vi "Galvo-Control-V3.vi"() -> ()   [LabVIEW 2024]
uses:
  <vilib>/DAQmx/write.llb/DAQmx Write (Analog 2D DBL NChan NSamp).vi
  <vilib>/DAQmx/write.llb/DAQmx Write (Analog 1D DBL NChan 1Samp).vi
  <vilib>/DAQmx/create/channels.llb/DAQmx Create Channel (AO-Voltage-Basic).vi
  <vilib>/DAQmx/miscellaneous.llb/DAQmx Fill In Error Info.vi
  <vilib>/measure/NI_MABase.lvlib
panel:
  out "Y MIN":dbl
  out "Y MAX":dbl
  out "X MIN":dbl
  out "X MAX":dbl
  out "Waveform Chart":waveform(dbl)(graph)
  out "Waveform Chart 2":waveform(dbl)(graph)
  in  "offset X":dbl format="%0.2p"
  in  "amplitude X":dbl=1.0 format="%0.2p"
  in  "phase":dbl format="%.2p"
  in  "amplitude Y":dbl=1.0 format="%0.2p"
  in  "phase 2":dbl format="%.2p"
  in  "offset Y":dbl format="%0.2p"
  in  "COMMENCE SCAN":bool
  in  "Y desired voltage step(V/100)":dbl=1.0 format="%#_13g"
  in  "X desired voltage step(V/100)":dbl=1.0 format="%#_13g"
  out "Virtual Y position":dbl(graph)
  out "virtual X position":dbl(graph)
  out "Y position":dbl
  out "X position.":dbl
  # "This VI is intended for the user to first define a\nrectangular region to scan, and then to commence\nthe scan at some desired resolution.\n\nthe resolution is defined using the voltage step controls\nat the bottom left region.\n\nthe amplitude and offset controls define the scan region"
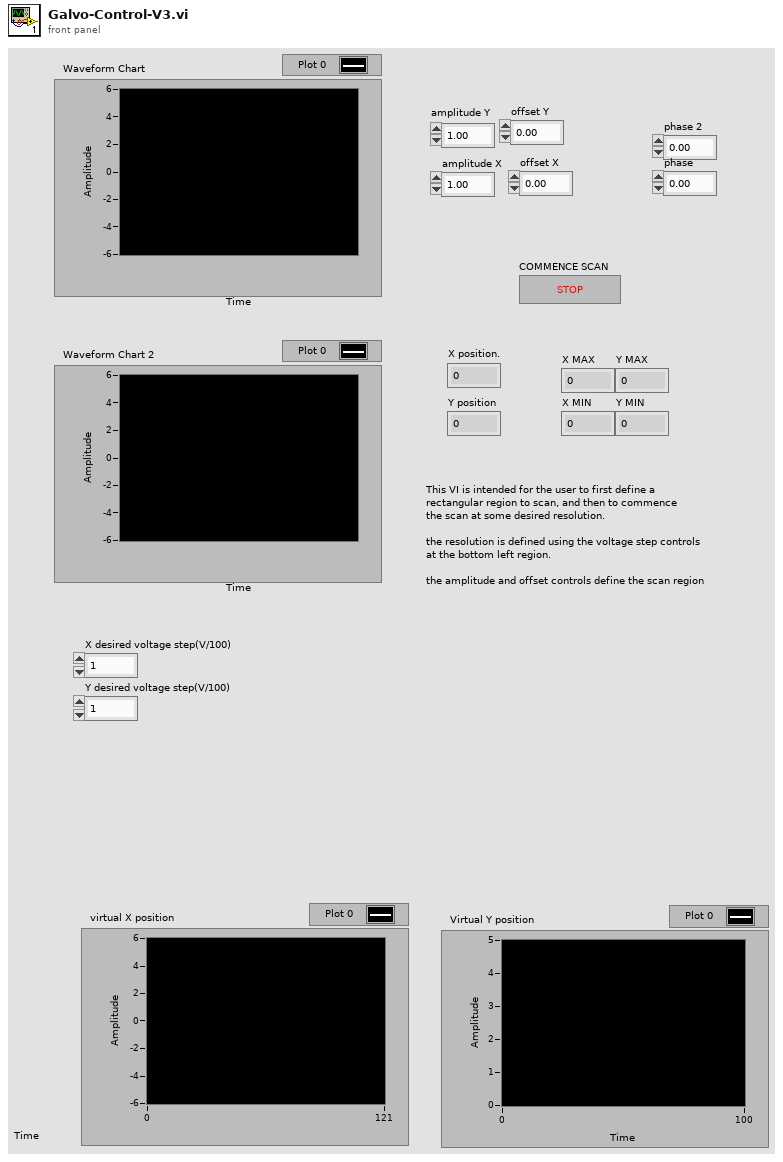
[diagram p1: front panel]
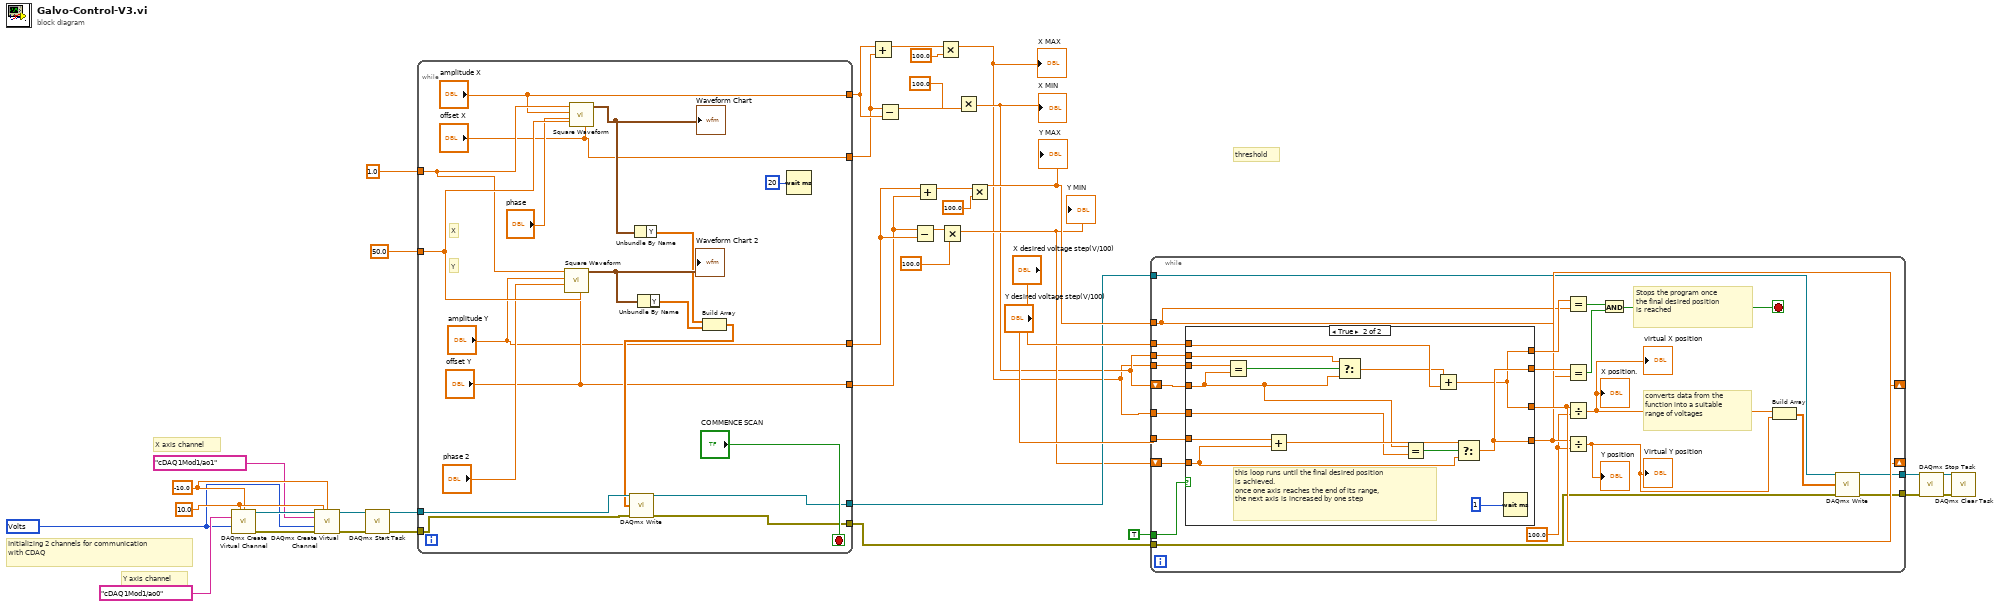
[diagram p0: block diagram]
diagram:
  w23 = 10348 items=["Volts"=10348, "From Custom Scale"=10065] ("units")
  w27 = 10.0 ("maximum value")
  w26 = -10.0 ("minimum value")
  # "Initializing 2 channels for communication\nwith CDAQ"
  # "X axis channel"
  # "Y axis channel"
  # "threshold"
  n1 = call-poly <vilib>:"DAQmx Create Virtual Channel.vi"("maximum value"=w27, "minimum value"=w26, "physical channels"=tag "cDAQ1Mod1/ao0", "units"=w23) -> ("task out"=w29:refnum<k21>, "error out"=w28:errorcluster)  [unwired: 10 in]
  n2 = call-poly <vilib>:"DAQmx Create Virtual Channel.vi"("task in"=w29, "maximum value"=w27, "minimum value"=w26, "physical channels"=tag "cDAQ1Mod1/ao1", "units"=w23, "error in"=w28) -> ("task out"=w22:refnum<k21>, "error out"=w21:errorcluster)  [unwired: 8 in]
  n3 = call <vilib>:"DAQmx Start Task.vi"("task/channels in"=w22, "error in"=w21) -> ("task out"=w20:refnum<k21>, "error out"=w19:errorcluster)  [unwired: 12 in]
  n4 = while {
    tunnel: 50.0 ("duty cycle (%)") -> [w57]
    tunnel: 1.0 ("frequency") -> [w56]
    tunnel: w20 -> [w51]
    tunnel: w19 -> [w50]
    tunnel: [w44] -> w15
    tunnel: [w43] -> w14
    tunnel: ["offset X"] -> w3
    tunnel: ["amplitude X"] -> w8
    tunnel: ["offset Y"] -> w1
    tunnel: ["amplitude Y"] -> w6
    stop <- "COMMENCE SCAN" stop-if-true
    # "Y"
    # "X"
    n5 = call <vilib>:"Square Waveform.vi"("duty cycle (%)"=w57, "offset"="offset Y", "phase"="phase 2", "amplitude"="amplitude Y", "frequency"=w56) -> ("signal out"=w49:waveform(dbl))  [unwired: 5 in, 1 out]
    "Waveform Chart 2" <- w49
    n6 = call <vilib>:"Square Waveform.vi"("duty cycle (%)"=w57, "offset"="offset X", "phase"="phase", "amplitude"="amplitude X", "frequency"=w56) -> ("signal out"=w48:waveform(dbl))  [unwired: 5 in, 1 out]
    "Waveform Chart" <- w48
    n7 = Unbundle By Name(w48) -> ("Y"=w47:dbl[])
    n8 = Unbundle By Name(w49) -> ("Y"=w46:dbl[])
    n9 = Build Array(w47, w46) -> (w45:dbl[][])
    n10 = call-poly <vilib>:"DAQmx Write.vi"("task/channels in"=w51, "data"=w45, "error in"=w50) -> ("task out"=w44:refnum<k21>, "error out"=w43:errorcluster)  [unwired: 10 in, 1 out]
    n11 = Wait (ms)(milliseconds to wait=u32 20) -> ()  [unwired: 1 out]
  }
  n12 = Add(x=w8, y=w3) -> (x+y=w4:dbl)
  n13 = Subtract(x=w3, y=w8) -> (x-y=w9:dbl)
  n14 = Subtract(x=w1, y=w6) -> (x-y=w7:dbl)
  n15 = Add(x=w6, y=w1) -> (x+y=w2:dbl)
  n16 = Multiply(x=w4, y=100.0) -> (x*y=w5:dbl)
  "X MAX" <- w5
  n17 = Multiply(x=w7, y=100.0) -> (x*y=w13:dbl)
  "Y MIN" <- w13
  n18 = Multiply(x=w9, y=100.0) -> (x*y=w11:dbl)
  "X MIN" <- w11
  n19 = Multiply(x=w2, y=100.0) -> (x*y=w17:dbl)
  "Y MAX" <- w17
  n20 = while {
    shift-right: [w73] -> _
    shift-left: w11 -> [w81]
    shift-right: [w72] -> _
    shift-left: w13 -> [w80]
    tunnel: TRUE -> [w76]
    tunnel: [w67] -> w37
    tunnel: [w66] -> w36
    tunnel: w15 -> [w65]
    tunnel: w14 -> [w64]
    tunnel: "Y desired voltage step(V/100)" -> [w63]
    tunnel: "X desired voltage step(V/100)" -> [w62]
    tunnel: w5 -> [w61]
    tunnel: w5 -> [w60]
    tunnel: w17 -> [w59]
    tunnel: w11 -> [w58]
    stop <- w77 stop-if-true
    w71 = 100.0 ("x")
    # "converts data from the\nfunction into a suitable \nrange of voltages"
    # "Stops the program once\nthe final desired position \nis reached"
    n21 = case shown="True" w76 {
      tunnel: w81 -> [_ w82]
      tunnel: [_ w90] -> w73
      tunnel: w80 -> [_ w92]
      tunnel: [_ w91] -> w72
      tunnel: [_ w90] -> w75
      tunnel: [_ w91] -> w74
      tunnel: w63 -> [_ w88]
      tunnel: w62 -> [_ w87]
      tunnel: w61 -> [_ w86]
      tunnel: w60 -> [_ w85]
      tunnel: w58 -> [_ w84]
      frame False {
      }
      frame True {
        # "this loop runs until the final desired position\nis achieved.\nonce one axis reaches the end of its range,\nthe next axis is increased by one step"
        n22 = Equal?(x=w86, y=w82) -> (x = y?=w95:bool)
        n23 = Add(x=w88, y=w92) -> (x+y=w93:dbl)
        n24 = Select(t=w84, s=w95, f=w82) -> (s? t:f=w83:dbl)
        n25 = Equal?(x=w82, y=w85) -> (x = y?=w94:bool)
        n26 = Add(x=w83, y=w87) -> (x+y=w90:dbl)
        n27 = Select(t=w93, s=w94, f=w92) -> (s? t:f=w91:dbl)
        n28 = Wait (ms)(milliseconds to wait=u32 1) -> ()  [unwired: 1 out]
      }
    }
    n29 = Equal?(x=w75, y=w59) -> (x = y?=w79:bool)
    n30 = Equal?(x=w74, y=w59) -> (x = y?=w78:bool)
    n31 = Divide(x=w73, y=w71) -> (x/y=w69:dbl)
    "X position." <- w69
    "virtual X position" <- w69
    n32 = Divide(x=w72, y=w71) -> (x/y=w70:dbl)
    "Y position" <- w70
    "Virtual Y position" <- w70
    n33 = And(x=w79, y=w78) -> (x .and. y?=w77:bool)
    n34 = Build Array(w69, w70) -> (w68:dbl[])
    n35 = call-poly <vilib>:"DAQmx Write.vi"("task/channels in"=w65, "data"=w68, "error in"=w64) -> ("task out"=w67:refnum<k21>, "error out"=w66:errorcluster)  [unwired: 10 in, 1 out]
  }
  n36 = call <vilib>:"DAQmx Stop Task.vi"("task/channels in"=w37, "error in"=w36) -> ("task out"=w35:refnum<k21>, "error out"=w34:errorcluster)  [unwired: 12 in]
  n37 = call <vilib>:"DAQmx Clear Task.vi"("task in"=w35, "error in"=w34) -> ()  [unwired: 13 in, 1 out]
